vi "Agilent PSG MXG Series BERT Using Custom Digital Modulation.vi"() -> ()   [LabVIEW 2018]
doc: "This example shows how to take a BERT measurement using Custom Digital Modulation.\n\n<B>Note:</B>\nIt is only valid in N5172B/82B that installs with <B>Option UN7</B> and <B>Option 431</B>."
uses:
  Agilent PSG MXG Series.lvlib
panel:
  in  "Aux IO Trigger Polarity (0: Positive)":i32(ring) items=["Positive", "Negative"]
  in  "Triggering Mode (0: Immediate)":i32(ring) items=["Immediate", "Key", "Ext", "Bus", "Aux I/O"]
  in  "Connector (4: Data Clock Out)":i32(ring)=4 items=["Burst Gate In", "Data Clock", "Data", "Symbol Sync", "Data Clock  Out", "Data Out", "Symbol Sync Out"]
  in  "Phase Polarity (0: Normal)":u16(ring) items=["Normal", "Inverted"]
  in  "I/Q Scaling (70 percent)":dbl=70.0
  in  "Symbol Rate (1.00000000E+06 sps)":dbl=1000000.0 format="%.8e"
  in  "Standard (0: None)":u16(ring) items=["None", "APCO 25 w/C4FM", "APCO 25 w/CQPSK", "Bluetooth", "CDPD"]
  in  "VISA resource name":refnum<visa-resource-name>
  # "(c) 2016 National Instruments.  ALL RIGHTS RESERVED."
  # "This example requires:\n1. N5102A is connected to the digital bus.\n2. The following connections on the signal generator's rear panel.\n       (1) DATA OUT (Aux I/O connector pin 33) to BER DATA IN (BNC connector labeled EVENT 1)\n       (2) DATA CLK OUT (Aux I/O connector pin 7) to BER CLK IN (BNC connector labeled BB TRIG1).\n3. This VI is only valid in N5172B/82B that installs with Option UN7 and Option 431."
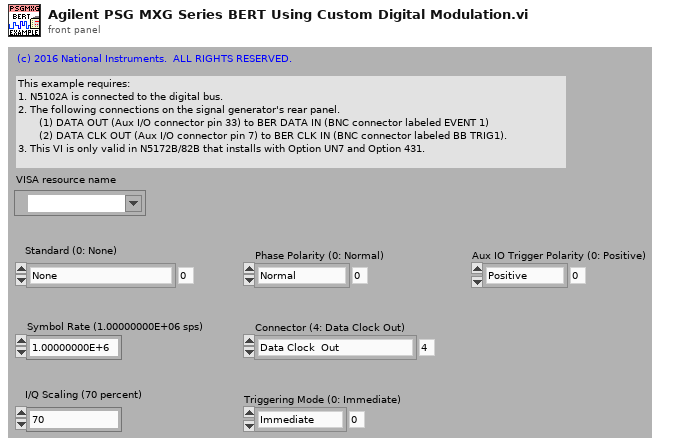
[diagram p1: front panel]
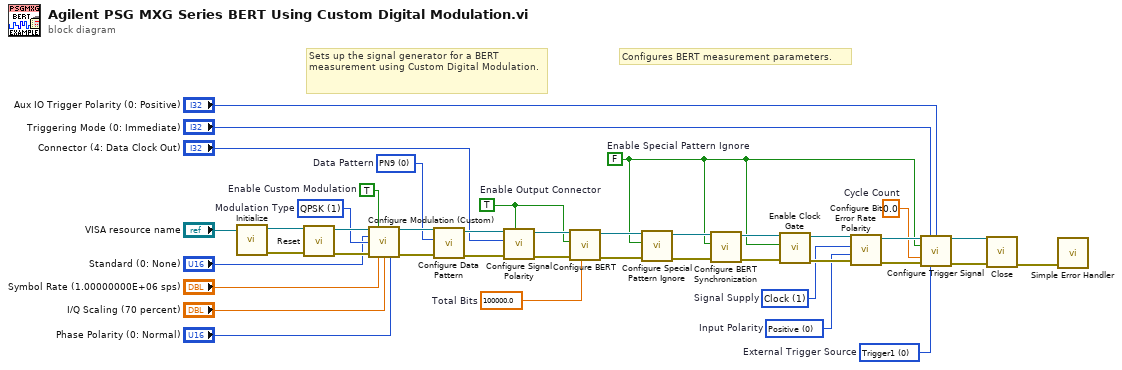
[diagram p0: block diagram]
diagram:
  w10 = 0 items=["Trigger1", "Trigger2", "Pulse"]  # External Trigger Source
  w12 = 0.0  # Cycle Count
  w15 = 0 items=["Positive", "Negative"]  # Input Polarity
  w16 = 1 items=["Gate", "Clock", "Data"]  # Signal Supply
  w11 = FALSE  # Enable Special Pattern Ignore
  w25 = 100000.0  # Total Bits
  w26 = TRUE  # Enable Output Connector
  w31 = u16 0 items=["PN9", "PN11", "PN15", "PN20", "PN23", "FIX4", "Select File", "External", "4 1's & 4 0's", "8 1's & 8 0's", "16 1's & 16 0's", "32 1's & 32 0's", "64 1's & 64 0's", "PRAM File"]  # Data Pattern
  w34 = TRUE  # Enable Custom Modulation
  w35 = u16 1 items=["BPSK", "QPSK", "IS-95 QPSK", "Gray Coded QPSK", "OQPSK", "IS-95 OQPSK", "pi/4 DQPSK", "8PSK", "16PSK", "D8PSK", "MSK", "2-Lvl FSK", "4-Lvl FSK", "8-Lvl FSK", "16-Lvl FSK", "C4FM", "4QAM", "16QAM", "32QAM", "64QAM", "128QAM", "256QAM", "User I/Q", "User FSK", "ASK", "UQPSK", "EDGE", "1024QAM", "VSA 16QAM", "VSA 32QAM", "VSA 64QAM", "VSA 128QAM", "VSA 256QAM", "VSA 512QAM", "VSA 1024QAM"]  # Modulation Type
  # "Configures BERT measurement parameters."
  # "Sets up the signal generator for a BERT measurement using Custom Digital Modulation."
  n1 = call "Initialize.vi"("VISA resource name"="VISA resource name") -> ("error out"=w38:errorcluster, "VISA resource name out"=w39:refnum<visa-resource-name>)  [unwired: 3 in, 6 out]
  n2 = call "Reset.vi"("error in (no error)"=w38, "VISA resource name"=w39) -> ("error out"=w36:errorcluster, "VISA resource name out"=w37:refnum<visa-resource-name>)  [unwired: 8 in]
  n3 = call "Configure Modulation (Custom).vi"("VISA resource name"=w37, "Enable Custom Modulation (T:Enable)"=w34, "Standard (0: None)"="Standard (0: None)", "Modulation Type (6: pi/4 DQPSK)"=w35, "error in (no error)"=w36, "Symbol Rate (24.3 ksps)"="Symbol Rate (1.00000000E+06 sps)", "I/Q Scaling (70 percent)"="I/Q Scaling (70 percent)", "Phase Polarity (0: Normal)"="Phase Polarity (0: Normal)") -> ("VISA resource name out"=w33:refnum<visa-resource-name>, "error out"=w32:errorcluster)  [unwired: 6 in]
  n4 = call "Configure Data Pattern.vi"("error in (no error)"=w32, "Data Pattern (4: PN23)"=w31, "VISA resource name"=w33) -> ("error out"=w29:errorcluster, "VISA resource name out"=w30:refnum<visa-resource-name>)  [unwired: 7 in]
  n5 = call "Configure Signal Polarity.vi"("Enable Output Connector (T: Enable)"=w26, "error in (no error)"=w29, "Connector (0: Burst Gate In connector)"="Connector (4: Data Clock Out)", "VISA resource name"=w30) -> ("error out"=w27:errorcluster, "VISA resource name out"=w28:refnum<visa-resource-name>)  [unwired: 6 in]
  n6 = call "Configure BERT.vi"("Total Bits (10000)"=w25, "error in (no error)"=w27, "Enable BERT (F: Disable)"=w26, "VISA resource name"=w28) -> ("error out"=w23:errorcluster, "VISA resource name out"=w24:refnum<visa-resource-name>)  [unwired: 6 in]
  n7 = call "Configure Special Pattern Ignore.vi"("error in (no error)"=w23, "Enable Special Pattern Ignore (F: Disable)"=w11, "VISA resource name"=w24) -> ("error out"=w21:errorcluster, "VISA resource name out"=w22:refnum<visa-resource-name>)  [unwired: 7 in]
  n8 = call "Configure BERT Synchronization.vi"("error in (no error)"=w21, "Enable Resynchronization (T: Enable)"=w11, "VISA resource name"=w22) -> ("error out"=w19:errorcluster, "VISA resource name out"=w20:refnum<visa-resource-name>)  [unwired: 7 in]
  n9 = call "Enable Clock Gate.vi"("error in (no error)"=w19, "Enable Gate (F: Disable)"=w11, "VISA resource name"=w20) -> ("error out"=w17:errorcluster, "VISA resource name out"=w18:refnum<visa-resource-name>)  [unwired: 7 in]
  n10 = call "Configure Bit Error Rate Polarity.vi"("error in (no error)"=w17, "Input Polarity (0: Positive)"=w15, "Signal Supply (0: Gate)"=w16, "VISA resource name"=w18) -> ("error out"=w14:errorcluster, "VISA resource name out"=w13:refnum<visa-resource-name>)  [unwired: 6 in]
  n11 = call "Configure Trigger Signal.vi"("VISA resource name"=w13, "Trigger Mode (1: Key)"="Triggering Mode (0: Immediate)", "Aux IO Trigger Polarity (0: Positive)"="Aux IO Trigger Polarity (0: Positive)", "Enable Trigger Delay (F: Disable)"=w11, "Cycle Count (1)"=w12, "error in (no error)"=w14, "External Trigger Source (0: Trigger1)"=w10) -> ("VISA resource name out"=w9:refnum<visa-resource-name>, "error out"=w8:errorcluster)  [unwired: 7 in]
  n12 = call "Close.vi"("error in (no error)"=w8, "VISA resource name"=w9) -> ("error out"=w40:errorcluster)  [unwired: 9 in]
  n13 = call <vilib>:"Simple Error Handler.vi"("error in (no error)"=w40) -> ()  [unwired: 4 in, 5 out]
